vi "Get CD Ref.vi"(8 "error in (no error)":errorcluster, 11 "Item Ref in":T1 format="%.0x") -> (0 "error out":errorcluster, 2 "CD Ref out":T1=18446744073709551615 format="%.0x", 3 "Item Ref out":T1 format="%.0x")   [LabVIEW 2011, in "Engine Sim System Explorer.lvlib"]
uses:
  Engine Sim System Explorer.lvlib
  <vilib>/NI Veristand/Custom Device API/Custom Device Item Ref.ctl
  Shared/Engine Simulation Global.vi
  <vilib>/NI Veristand/Custom Device API/Custom Device API.lvlib
  Engine Simulation Shared.lvlib
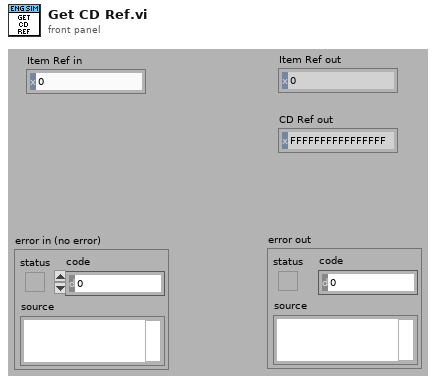
[diagram p1: front panel]
types:
  T1 = typedef "Custom Device API.lvlib/Custom Device Item Ref.ctl" = u64
  T2 = typedef "Custom Device API.lvlib/Custom Device Item Info.ctl" = cluster{"Name":string, "Is Channel":bool, "GUID":string}
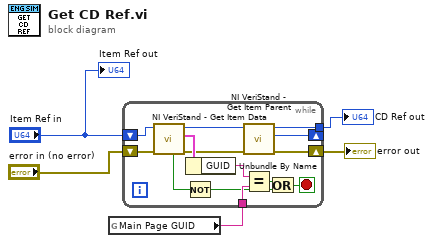
[diagram p0: block diagram]
diagram:
  n1 = global read "Engine Simulation Global.vi" "Main Page GUID"() -> (w5:string)
  n2 = while {
    shift-right: [w15] -> w2
    shift-left: "error in (no error)" -> [w14]
    shift-right: [w13] -> _
    shift-left: "Item Ref in" -> [w19]
    tunnel: [w12] -> w1
    tunnel: w5 -> [w10]
    stop <- w8 stop-if-true
    n3 = call <vilib>:"NI VeriStand - Get Item Data.vi"("error in (no error)"=w14, "Item Ref in"=w19) -> ("error out"=w16:errorcluster, "Item Info"=w17:T2, "Item Ref out"=w18:T1, "Found"=w7:bool)  [unwired: 6 in]
    n4 = Not(x=w7) -> (.not. x?=w6:bool)
    n5 = Unbundle By Name(w17) -> ("GUID"=w11:string)
    n6 = call <vilib>:"NI VeriStand - Get Item Parent.vi"("error in (no error)"=w16, "Item Ref in"=w18) -> ("error out"=w15:errorcluster, "Parent Ref"=w13:T1, "Item Ref out"=w12:T1)  [unwired: 6 in, 1 out]
    n7 = Equal?(x=w11, y=w10) -> (x = y?=w9:bool)
    n8 = Or(x=w9, y=w6) -> (x .or. y?=w8:bool)
  }
  "error out" <- w2
  "CD Ref out" <- w1
  "Item Ref out" <- "Item Ref in"
